vi "Handle Composition.vi"(8 "error in":errorcluster, 11 "cPAS Facade in":refnum<class "cPAS Facade.lvclass">) -> (0 "error out":errorcluster, 3 "cPAS Facade out":refnum<class "cPAS Facade.lvclass">)   [LabVIEW 2015, in "cPAS Facade.lvclass"]
uses:
  cPAS Facade.lvclass
  Reusable/GUI/Composition/GUI Composition.lvclass
  UIs.ctl
  Reusable/GUI/Facade/GUI Facade.lvclass/GUI Facade.ctl
  Reusable/GUI/Composition/GUI Composition.lvclass/GUI Composition.ctl
  Reusable/GUI/Facade/Accessors/Read GUIs.vi
  Reusable/GUI/Facade/Accessors/Read FP Refs.vi
  Reusable/GUI/Composition/Accessors/Write GUIs.vi
  Reusable/GUI/Composition/Accessors/Write Panel Refs.vi
  Reusable/GUI/Facade/Accessors/Write GUIs.vi
  Reusable/GUI/Facade/Accessors/Write FP Refs.vi
  Reusable/GUI/GUI.lvclass
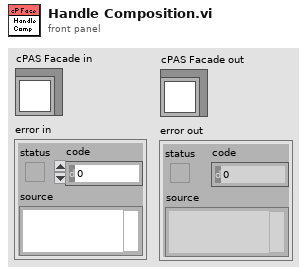
[diagram p1: front panel]
types:
  T1 = typedef "cPAS Facade.lvclass/UIs.ctl" = enum8{"PAS HF", "PAS Ctl", "PAS Der", "PAS HK", "Common", "Pcal", "CRD Ctl", "CRD RD", "CRD Der", "CRD HK", "Calibration", "CLAP", "Derived", "Housekeeping"}
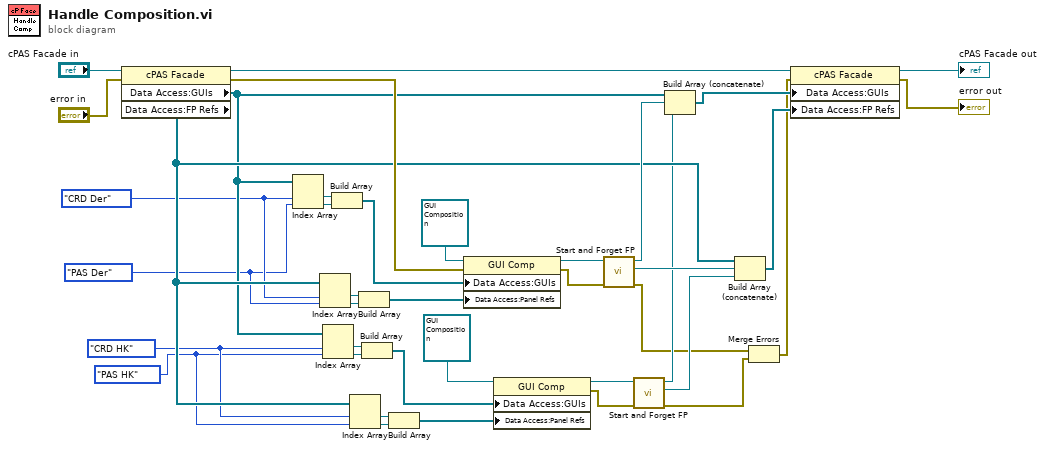
[diagram p0: block diagram]
diagram:
  w5 = UIs."CRD HK" ("UIs")
  w4 = UIs."PAS HK" ("UIs")
  w6 = UIs."PAS Der" ("UIs")
  w7 = UIs."CRD Der" ("UIs")
  n1 = property class="cPAS Facade"(reference="cPAS Facade in", error in="error in") -> (reference out=w27:refnum<class "cPAS Facade.lvclass">, error out=w33:errorcluster, "Data Access:GUIs"=w10:refnum<class "GUI.lvclass">[], "Data Access:FP Refs"=w11:refnum<vi>[])
  n2 = Index Array(array=w10, index #1=w7, index #2=w6) -> (element #1=w37:refnum<class "GUI.lvclass">, element #2=w36:refnum<class "GUI.lvclass">)
  n3 = Index Array(array=w11, index #1=w7, index #2=w6) -> (element #1=w29:refnum<vi>, element #2=w30:refnum<vi>)
  n4 = Index Array(array=w10, index #1=w5, index #2=w4) -> (element #1=w15:refnum<class "GUI.lvclass">, element #2=w16:refnum<class "GUI.lvclass">)
  n5 = Build Array(w37, w36) -> (w35:refnum<class "GUI.lvclass">[])
  n6 = Index Array(array=w11, index #1=w5, index #2=w4) -> (element #1=w20:refnum<vi>, element #2=w19:refnum<vi>)
  n7 = Build Array(w29, w30) -> (w28:refnum<vi>[])
  n8 = Build Array(w15, w16) -> (w17:refnum<class "GUI.lvclass">[])
  n9 = Build Array(w20, w19) -> (w12:refnum<vi>[])
  n10 = property class="GUI Comp"(reference=refnum<class "GUI Composition.lvclass"> refnum ("GUI Composition.lvclass"), error in=w33, "Data Access:GUIs"=w35, "Data Access:Panel Refs"=w28) -> (reference out=w38:refnum<class "GUI Composition.lvclass">, error out=w31:errorcluster)
  n11 = property class="GUI Comp"(reference=refnum<class "GUI Composition.lvclass"> refnum ("GUI Composition.lvclass"), "Data Access:GUIs"=w17, "Data Access:Panel Refs"=w12) -> (reference out=w14:refnum<class "GUI Composition.lvclass">, error out=w18:errorcluster)  [unwired: 1 in]
  n12 = call "Start and Forget FP.vi"("error in"=w31, "GUI in"=w38) -> ("error out"=w3:errorcluster, "UI Ref"=w21:refnum<vi>, "GUI out"=w26:refnum<class "GUI Composition.lvclass">)  [unwired: 6 in, 1 out]
  n13 = call "Start and Forget FP.vi"("error in"=w18, "GUI in"=w14) -> ("error out"=w2:errorcluster, "UI Ref"=w9:refnum<vi>, "GUI out"=w8:refnum<class "GUI Composition.lvclass">)  [unwired: 6 in, 1 out]
  n14 = Build Array (concatenate)(w10, w26, w8) -> (w23:refnum<class "GUI.lvclass">[])
  n15 = Build Array (concatenate)(w11, w21, w9) -> (w22:refnum<vi>[])
  n16 = Merge Errors(w3, w2) -> (w1:errorcluster)
  n17 = property class="cPAS Facade"(reference=w27, error in=w1, "Data Access:GUIs"=w23, "Data Access:FP Refs"=w22) -> (reference out=→"cPAS Facade out":refnum<class "cPAS Facade.lvclass">, error out=→"error out":errorcluster)
